vi "Part 1.vi"(11 "Input":string) -> (3 "Output":i64)   [LabVIEW 2021]
uses:
  <userlib>/_OpenG.lib/string/string.llb/Convert EOLs (String)__ogtk.vi
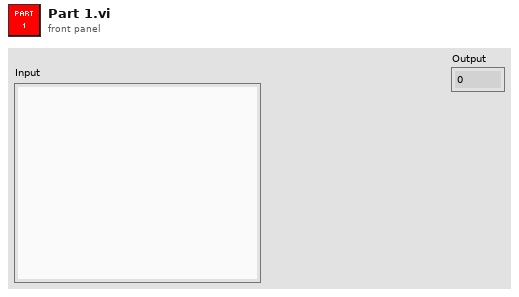
[diagram p1: front panel]
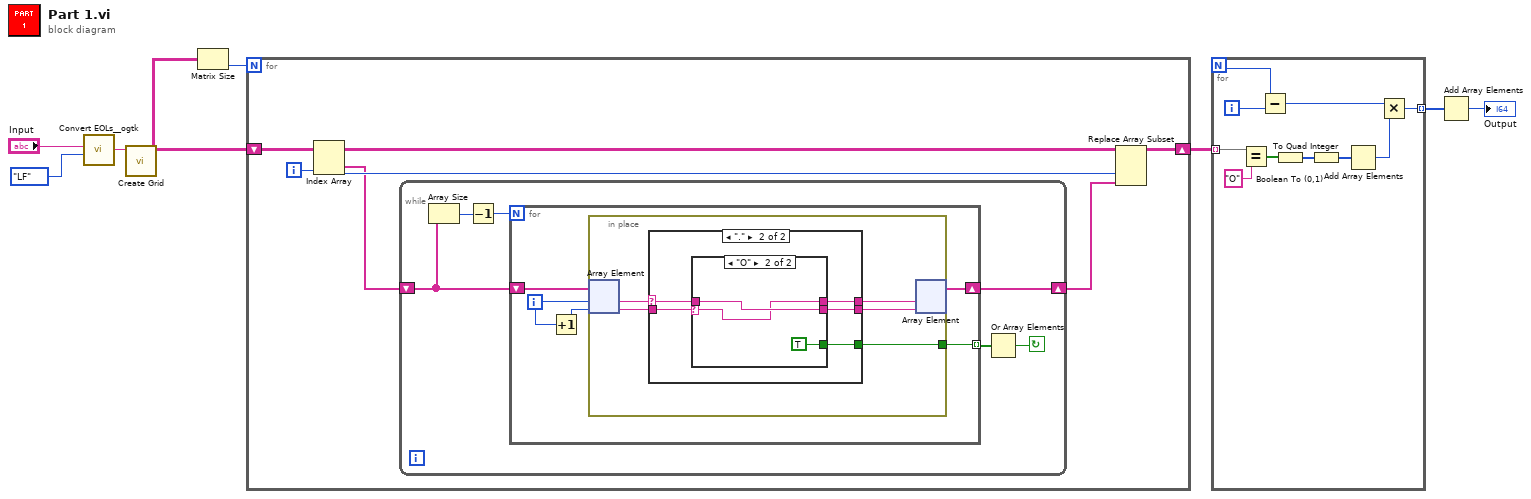
[diagram p0: block diagram]
diagram:
  n1 = call-poly <userlib>:"Convert EOLs__ogtk.vi"("Convert to:"=enum16{"CR", "LF", "CRLF"}."LF", "String in"="Input") -> ("String out"=w6:string)  [unwired: 9 in]
  n2 = call "Create Grid.vi"("String"=w6) -> ("Array"=w4:string[][])  [unwired: 10 in]
  n3 = Matrix Size(0:w4) -> (2:w5:i32)  [unwired: 1 out]
  n4 = for {
    N: w5 -> [_]
    shift-right: [w12] -> w3
    shift-left: w4 -> [w13]
    i -> [w11]
    n5 = Index Array(array=w13, index (col)=w11) -> (element=w10:string[])  [unwired: 1 in]
    n6 = while {
      shift-right: [w17] -> w9
      shift-left: w10 -> [w16]
      stop <- w14 continue-if-true
      n7 = Array Size(array=w16) -> (size(s)=w19:i32)
      n8 = Decrement(x=w19) -> (x-1=w18:i32)
      n9 = for {
        N: w18 -> [_]
        shift-right: [w23] -> w17
        shift-left: w16 -> [w24]
        tunnel: [w20] -> w15 mode=indexing
        i -> [w21]
        n10 = Increment(x=w21) -> (x+1=w22:i32)
        n11 = in-place {
          in-place-border: [w25] -> w20
          n12 = in-place-array #1(w24, w21, w22) -> (w29:string, w28:string)
          n13 = case shown="\".\"" w29 {
            selector: w29 -> [w31 w34]
            tunnel: w28 -> [w30 w36]
            tunnel: [w31 w35] -> w27
            tunnel: [w30 w33] -> w26
            tunnel: [_ w32] -> w25
            frame Default {
            }
            frame "." {
              n14 = case shown="\"O\"" w36 {
                selector: w36 -> [w37 w40]
                tunnel: [w38 w40] -> w35
                tunnel: w34 -> [w38 w41]
                tunnel: [w37 w41] -> w33
                tunnel: [_ TRUE] -> w32
                frame Default {
                }
                frame "O" {
                }
              }
            }
          }
          n15 = in-place-array #1(w27, w26) -> (w23:string[])  [unwired: 2 out]
        }
      }
      n16 = Or Array Elements(Boolean array=w15) -> (logical OR=w14:bool)
    }
    n17 = Replace Array Subset(array=w13, new element=w9, index (col)=w11) -> (w12:string[][])  [unwired: 1 in]
  }
  n18 = for {
    N -> [w50]
    tunnel: w3 -> [w48] mode=indexing
    tunnel: [w43] -> w2 mode=indexing
    i -> [w51]
    n19 = Equal?(x=w48, y="O") -> (x = y?=w46:bool[])
    n20 = Subtract(x=w50, y=w51) -> (x-y=w49:i32)
    n21 = Boolean To (0,1)(Boolean=w46) -> (0, 1=w45:i16[])
    n22 = To Quad Integer(1:w45) -> (0:w42:i64[])
    n23 = Add Array Elements(numeric array=w42) -> (sum=w44:i64)
    n24 = Multiply(x=w49, y=w44) -> (x*y=w43:i64)
  }
  n25 = Add Array Elements(numeric array=w2) -> (sum=→"Output":i64)
